vi "初始化数组.vi"() -> ()   [LabVIEW 2018]
panel:
  out "数组":dbl[][](array[numeric])
  in  "维数大小 列":i32
  in  "维数大小 行":i32
  in  "元素":dbl
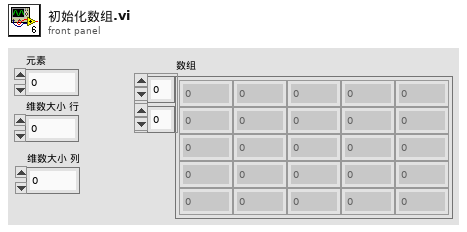
[diagram p1: front panel]
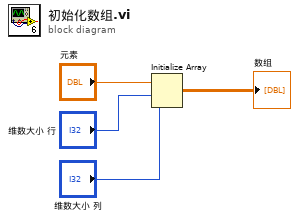
[diagram p0: block diagram]
diagram:
  n1 = Initialize Array("元素", "维数大小 行", "维数大小 列") -> (→"数组":dbl[][])
